vi "Control Grouping.vi"() -> ()   [LabVIEW 2019, in "LSS.lvlib"]
doc: "This simple example demonstrates what can be done by grouping multiple controls together while setting their properties. All properties applied to a group will be applied to all objects of that group that share the parcitular property being set. For example, if \"disable-state:true\" were sent to group1, all objects of group one would be disabled regardless of type."
uses:
  LSS.lvlib
panel:
  out "Explanation":string="Run program then click controls within the style control box to see the effect of grouping controls."
  in  "Color Group2":u32(colorbox)=12114431
  in  "Disable Group2":bool
  in  "Group2 Button3":bool
  in  "Group2 Button2":bool
  in  "Group2 Button1":bool
  out "Benchmark Operation Time (seconds)":dbl
  in  "Color Group1":u32(colorbox)=10551268
  in  "Disable Group1":bool
  in  "Tab Control":enum32{"One", "Two", "Three"}(tab)
  in  "Group1 String":string
  in  "Group2 Tab String":string
  in  "Group2 String":string
  in  "Group1 Boolean":bool
  # "Style Controls"
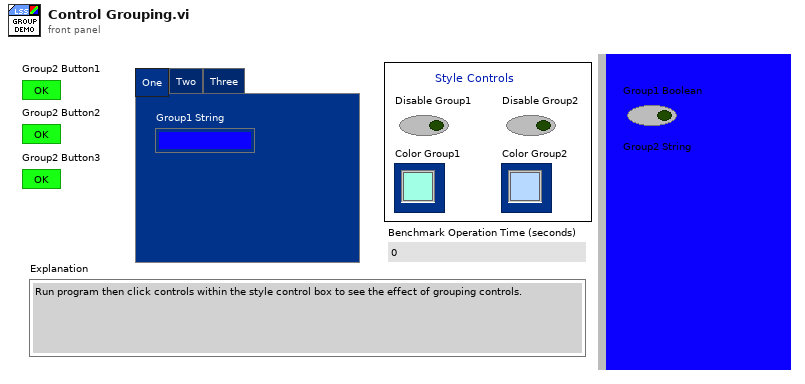
[diagram p1: front panel]
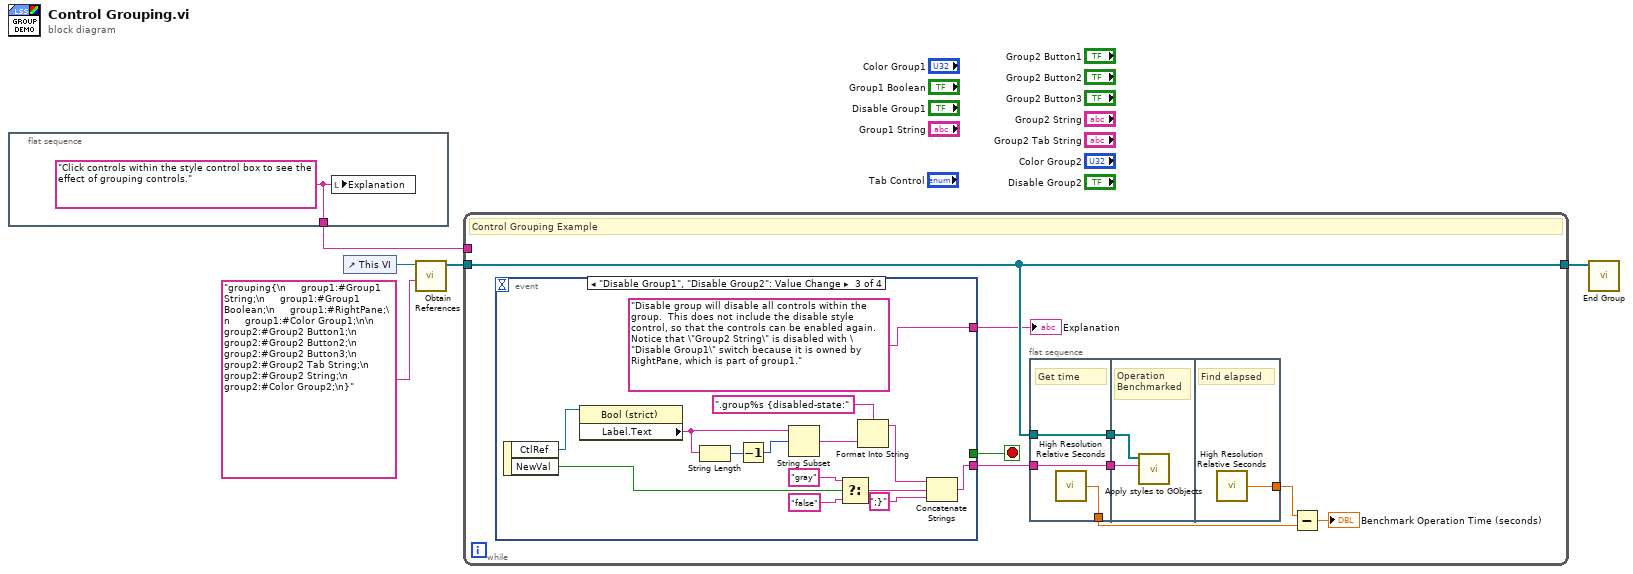
[diagram p0: block diagram]
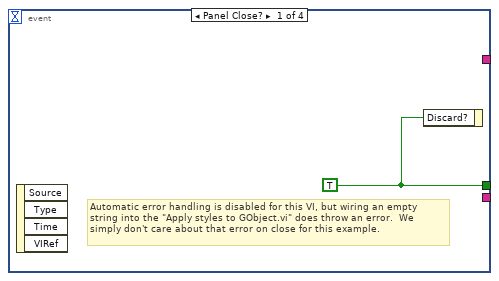
[diagram p2: hidden frame]
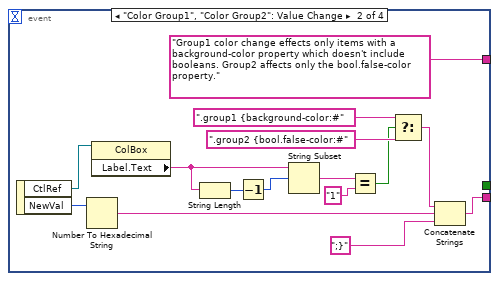
[diagram p3: hidden frame]
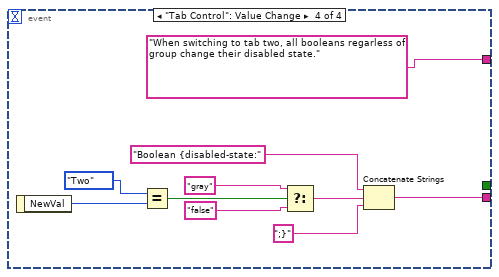
[diagram p4: hidden frame]
diagram:
  n1 = flat-sequence {
    tunnel: [w6] -> w2
    frame #0 {
      w6 = "Click controls within the style control box to see the effect of grouping controls." ("Explanation")
      n2 = local write "Explanation"(w6) -> ()
    }
  }
  n3 = control-ref of="This VI"() -> (w5:refnum<vi>)
  n4 = call "Obtain References.vi"("grouping"="grouping{\n     group1:#Group1 String;\n     group1:#Group1 Boolean;\n     group1:#RightPane;\n     group1:#Color Group1;\n\n     group2:#Group2 Button1;\n     group2:#Group2 Button2;\n     group2:#Group2 Button3;\n     group2:#Group2 Tab String;\n     group2:#Group2 String;\n     group2:#Color Group2;\n}" ("Tag Name"), "VI in"=w5) -> ("Front Panel Objects"=w4:refnum<vi>[])  [unwired: 8 in, 1 out]
  n5 = while {
    tunnel: w4 -> [w8]
    tunnel: [w8] -> w3
    tunnel: w2 -> [_]
    stop <- w15 stop-if-true
    # "Control Grouping Example"
    n6 = event shown="[2] \"Disable Group1\", \"Disable Group2\": Value Change" {
      selector: _ -> [_ _ _ _]
      dyn-events: _ -> [_ _ _ _]
      timeout: _ -> [_ _ _ _]
      tunnel: [w22 _ _ _] -> w15
      tunnel: [_ w34 w46 w54] -> w9
      tunnel: [_ "Group1 color change effects only items with a background-color property which doesn't include booleans. Group2 affects only the bool.false-color property." ("Explanation") "Disable group will disable all controls within the group.  This does not include the disable style control, so that the controls can be enabled again.  Notice that \"Group2 String\" is disabled with \"Disable Group1\" switch because it is owned by RightPane, which is part of group1." ("Explanation") "When switching to tab two, all booleans regarless of group change their disabled state." ("Explanation")] -> w7
      event Panel Close? {
        w22 = TRUE ("Discard?")
        # "Automatic error handling is disabled for this VI, but wiring an empty\nstring into the \"Apply styles to GObject.vi\" does throw an error.  We\nsimply don't care about that error on close for this example."
        n7 = event-data() -> ()  [unwired: 1 in, 4 out]
        n8 = event-data("Discard?"=w22) -> ()  [unwired: 1 in, 1 out]
      }
      event "Color Group1", "Color Group2": Value Change {
        n9 = event-data() -> ("CtlRef"=w30:refnum<vi>, "NewVal"=w36:u32)  [unwired: 1 in]
        n10 = Number To Hexadecimal String(2:w36) -> (0:w35:string)  [unwired: 1 in]
        n11 = property class="ColBox"(reference=w30) -> ("Label.Text"=w33:string)  [unwired: 1 in, 2 out]
        n12 = String Length(string=w33) -> (length=w32:i32)
        n13 = Decrement(x=w32) -> (x-1=w31:i32)
        n14 = String Subset(string=w33, offset (0)=w31) -> (substring=w27:string)  [unwired: 1 in]
        n15 = Equal?(x=w27, y="1") -> (x = y?=w25:bool)
        n16 = Select(t=".group1 {background-color:#" ("CSS in"), s=w25, f=".group2 {bool.false-color:#" ("CSS in")) -> (s? t:f=w24:string)
        n17 = Concatenate Strings(w24, w35, ";}" ("string")) -> (w34:string)
      }
      event "Disable Group1", "Disable Group2": Value Change {
        n18 = event-data() -> ("CtlRef"=w45:refnum<vi>, "NewVal"=w50:bool)  [unwired: 1 in]
        n19 = property class="Bool (strict)"(reference=w45) -> ("Label.Text"=w42:string)  [unwired: 1 in, 2 out]
        n20 = String Length(string=w42) -> (length=w41:i32)
        n21 = Decrement(x=w41) -> (x-1=w40:i32)
        n22 = String Subset(string=w42, offset (0)=w40) -> (substring=w39:string)  [unwired: 1 in]
        n23 = Select(t="gray" ("CSS in"), s=w50, f="false" ("CSS in")) -> (s? t:f=w49:string)
        n24 = Format Into String(format string=".group%s {disabled-state:" ("CSS in"), w39) -> (resulting string=w43:string)  [unwired: 2 in, 1 out]
        n25 = Concatenate Strings(w43, w49, ";}" ("string")) -> (w46:string)
      }
      event "Tab Control": Value Change {
        n26 = event-data() -> ("NewVal"=w59:enum32{"One", "Two", "Three"})  [unwired: 1 in]
        n27 = Equal?(x=enum32{"One", "Two", "Three"}."Two", y=w59) -> (x = y?=w55:bool)
        n28 = Select(t="gray" ("CSS in"), s=w55, f="false" ("CSS in")) -> (s? t:f=w58:string)
        n29 = Concatenate Strings("Boolean {disabled-state:" ("CSS in"), w58, ";}" ("string")) -> (w54:string)
      }
    }
    "Explanation" <- w7
    n30 = flat-sequence {
      tunnel: w8 -> [w17]
      tunnel: w9 -> [w18]
      tunnel: [w18] -> w14
      tunnel: [w17] -> w13
      tunnel: [w16] -> w12
      tunnel: w14 -> [w20]
      tunnel: w13 -> [w19]
      tunnel: [w21] -> w11
      frame #0 {
        # "Get time"
        n31 = call <vilib>:"High Resolution Relative Seconds.vi"() -> ("relative seconds"=w16:dbl)
      }
      frame #1 {
        # "Operation\nBenchmarked"
        n32 = call "Apply styles to GObjects.vi"("Style Sheet"=w20, "Front Panel Objects"=w19) -> ()  [unwired: 8 in, 2 out]
      }
      frame #2 {
        # "Find elapsed"
        n33 = call <vilib>:"High Resolution Relative Seconds.vi"() -> ("relative seconds"=w21:dbl)
      }
    }
    n34 = Subtract(x=w11, y=w12) -> (x-y=→"Benchmark Operation Time (seconds)":dbl)
  }
  n35 = call "End Group.vi"("Group Item References"=w3) -> ()  [unwired: 10 in, 1 out]
